vi "3Vote.vi"(10 "input":bool) -> (2 "output":bool)   [LabVIEW 2010, in "kevLib2010.lvlib"]
uses:
  kevLib2010.lvlib
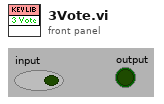
[diagram p1: front panel]
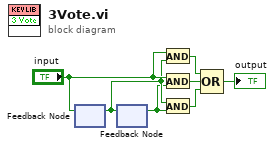
[diagram p0: block diagram]
diagram:
  n1 = feedback-in #1("input") -> ()
  n2 = feedback #1() -> (w2:bool)  [unwired: 1 out]
  n3 = feedback-in #2(w2) -> ()
  n4 = feedback #2() -> (w1:bool)  [unwired: 1 out]
  n5 = And(x="input", y=w2) -> (x .and. y?=w7:bool)
  n6 = And(x="input", y=w1) -> (x .and. y?=w6:bool)
  n7 = And(x=w2, y=w1) -> (x .and. y?=w5:bool)
  n8 = Compound Arithmetic op=OR(w7, w6, w5) -> (→"output":bool)
